vi "G#Object_GetEvent.vi"(1 "create if needed (T)":bool=TRUE, 2 "force create (F)":bool, 5 "error in (no error)":errorcluster) -> (15 "G# event":refnum<user-event>, 16 "created new":bool, 17 "valid":bool, 18 "event owner":string, 19 "error out":errorcluster)   [LabVIEW 2020, in "G#Object.lvclass"]
doc: "Returns the event used by the G#Object kernel to indicate that a new object has been created or has been deleted. This event is used by the debugger, but could be used by anyone."
uses:
  G#Object.lvclass
  utils/G#Object_Event.ctl
  utils/G#Object_EventType.ctl
  utils/G#Object_ObjectInfoType.ctl
  utils/G#Object_CreateMethod.ctl
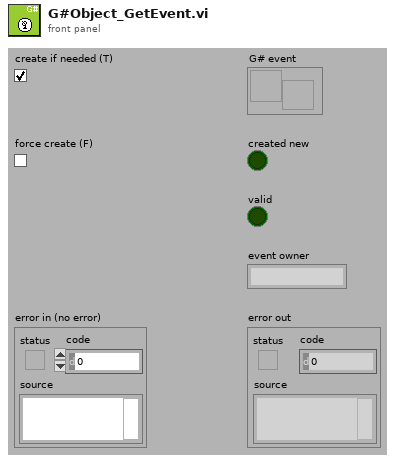
[diagram p1: front panel]
types:
  T1 = typedef "G#Object.lvclass/G#Object_Event.ctl" = cluster{"EventType":T2, "ObjectInfo":T3, "Ref":refnum<class "G#Object.lvclass">, "Time Stamp":timestamp, "LogText":string, "Parameters":variant[]}
  T2 = typedef "G#Object.lvclass/G#Object_EventType.ctl" = enum16{"Created new", "Looked up existing", "Deleted", "Forced delete", "Not deleted", "Garbage collected", "Cleared", "User", "Error", "External create object", "External create class attributes", "Created class attributes", "Run constructor", "Run constructor done", "Run open method", "Run open method done"}
  T3 = typedef "G#Object.lvclass/G#Object_ObjectInfoType.ctl" = cluster{"ObjectName":string, "ObjectID":u32, "Users":i32, "Counter":bool, "AttributeRefs":u32[], "FullClassName":string, "ClassName":string, "CreateMethod":T4, "GenericDestructorExists":bool, "Owner":string}
  T4 = typedef "G#Object.lvclass/G#Object_CreateMethod.ctl" = enum16{"Create", "Create or look up existing", "Look up existing"}
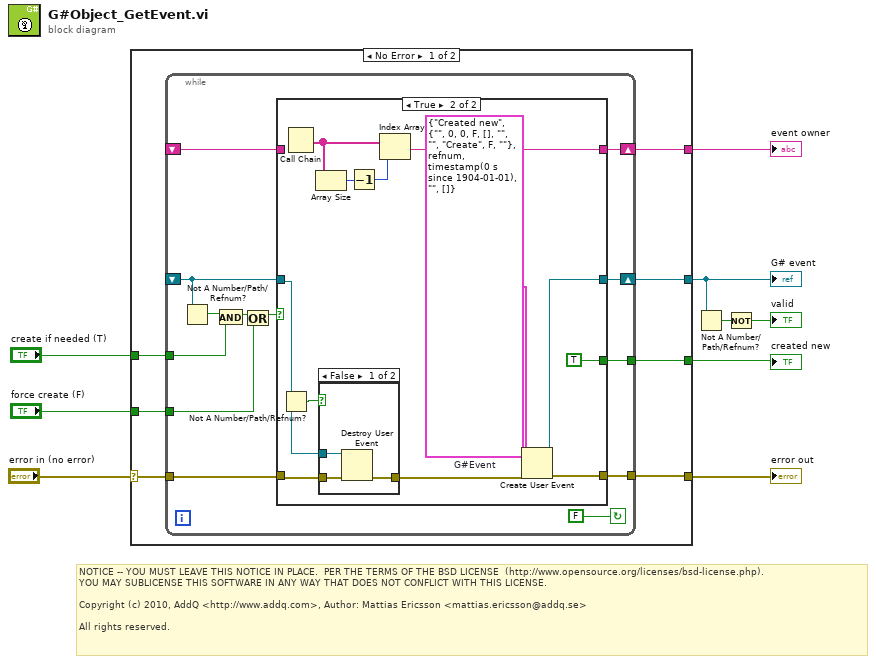
[diagram p0: block diagram]
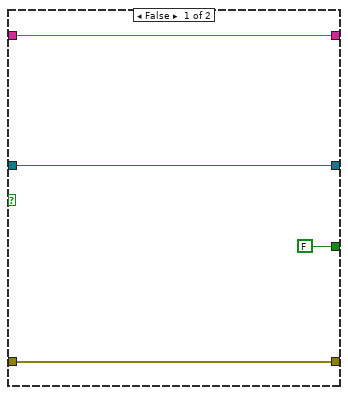
[diagram p2: hidden frame]
diagram:
  # "NOTICE -- YOU MUST LEAVE THIS NOTICE IN PLACE.  PER THE TERMS OF THE BSD LICENSE  (http://www.opensource.org/licenses/bsd-license.php).\nYOU MAY SUBLICENSE THIS SOFTWARE IN ANY WAY THAT DOES NOT CONFLICT WITH THIS LICENSE.\n\nCopyright (c) 2010, AddQ <http://www.addq.com>, Author: Mattias Ericsson <mattias.ericsson@addq.se>\n\nAll rights reserved."
  n1 = case shown="No Error" "error in (no error)" {
    selector: "error in (no error)" -> [w16 w50]
    tunnel: [w15 w50] -> w8
    tunnel: [w14 _] -> w6
    tunnel: "create if needed (T)" -> [w13 _]
    tunnel: [w12 _] -> w2
    tunnel: [w11 _] -> w3
    tunnel: "force create (F)" -> [w10 _]
    frame No Error {
      n2 = while {
        tunnel: w16 -> [w28]
        shift-right: [w27] -> w14
        shift-left: _ -> [w25]
        tunnel: [w26] -> w15
        tunnel: w13 -> [w23]
        shift-right: [w22] -> w12
        shift-left: _ -> [w21]
        tunnel: [w20] -> w11
        tunnel: w10 -> [w17]
        stop <- FALSE continue-if-true
        n3 = Not A Number/Path/Refnum?(number/path/refnum=w25) -> (NaN/Path/Refnum?=w24:bool)
        n4 = And(x=w24, y=w23) -> (x .and. y?=w18:bool)
        n5 = Or(x=w18, y=w17) -> (x .or. y?=w19:bool)
        n6 = case shown="True" w19 {
          tunnel: w28 -> [w32 w41]
          tunnel: [w33 w45] -> w27
          tunnel: [w32 w44] -> w26
          tunnel: w25 -> [w33 w38]
          tunnel: [w31 w34] -> w22
          tunnel: w21 -> [w31 _]
          tunnel: [FALSE TRUE] -> w20
          frame False {
          }
          frame True {
            w43 = T1 {"EventType"=enum."Created new", "ObjectInfo"={"ObjectName"="", "ObjectID"=0, "Users"=0, "Counter"=FALSE, "AttributeRefs"=[], "FullClassName"="", "ClassName"="", "CreateMethod"=enum."Create", "GenericDestructorExists"=FALSE, "Owner"=""}, "Ref"=refnum, "Time Stamp"=timestamp(0 s since 1904-01-01), "LogText"="", "Parameters"=[]}  # G#Event
            n7 = Not A Number/Path/Refnum?(number/path/refnum=w38) -> (NaN/Path/Refnum?=w40:bool)
            n8 = Call Chain() -> (call chain=w37:string[])
            n9 = Array Size(array=w37) -> (size(s)=w36:i32)
            n10 = case shown="False" w40 {
              tunnel: w41 -> [w48 w49]
              tunnel: [w47 w49] -> w39
              tunnel: w38 -> [w46 _]
              frame False {
                n11 = Destroy User Event(user event=w46, error in=w48) -> (error out=w47:errorcluster)
              }
              frame True {
              }
            }
            n12 = Decrement(x=w36) -> (x-1=w35:i32)
            n13 = Index Array(array=w37, index=w35) -> (element=w34:string)
            n14 = Create User Event(user event datatype=w43, error in=w39) -> (user event=w45:refnum<user-event>, error out=w44:errorcluster)
          }
        }
      }
    }
    frame Error {
    }
  }
  "error out" <- w8
  "G# event" <- w6
  "created new" <- w3
  "event owner" <- w2
  n15 = Not A Number/Path/Refnum?(number/path/refnum=w6) -> (NaN/Path/Refnum?=w5:bool)
  n16 = Not(x=w5) -> (.not. x?=→"valid":bool)
